vi "Add Compane.vi"(6 "Variant in":variant, 7 "Shift Pressed?":bool, 8 "error in (no error)":errorcluster, 10 "QD Combo Box Ref":refnum<vi>, 11 "QD Launch VI Ref":refnum<vi>) -> (0 "error out":errorcluster, 4 "Variant out":variant)   [LabVIEW 2015]
doc: "Add Control terminal to conpane.\n\nDefault Shortcut - [G]"
uses:
  <vilib>/Utility/config.llb/Read Key (String).vi
  <vilib>/Utility/config.llb/NI_LVConfig.lvlib
panel:
  # "Do not change the connector pane of this VI.\n\nSee the block diagram for directions on how to use this template."
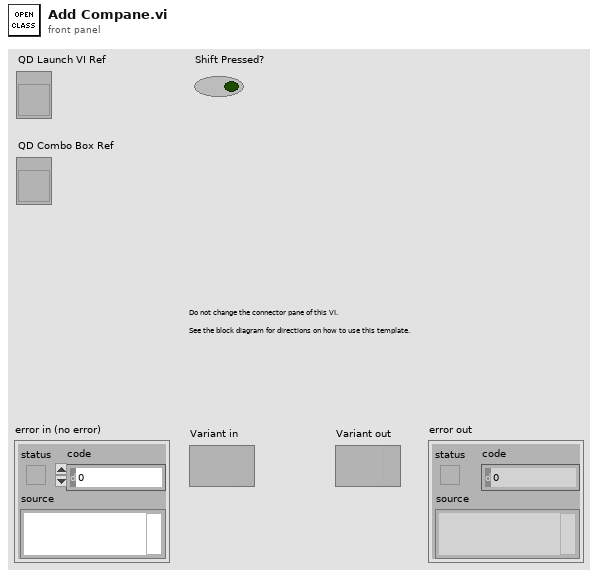
[diagram p1: front panel]
types:
  T1 = typedef "NI_LVConfig.lvlib/Config Data RefNum.ctl" = refnum<k1>
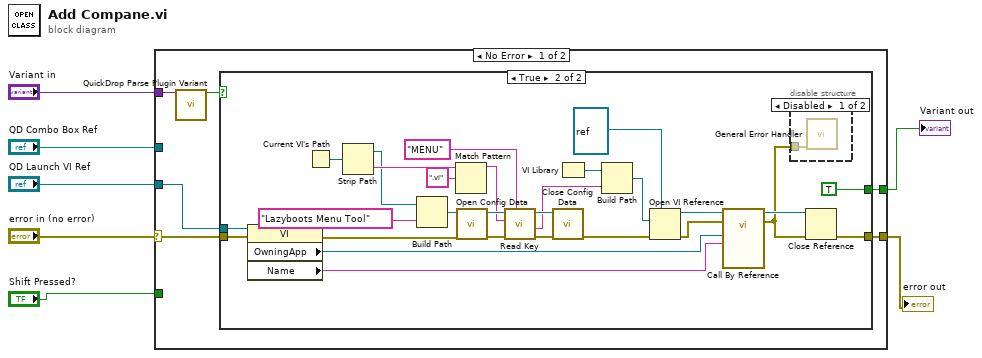
[diagram p0: block diagram]
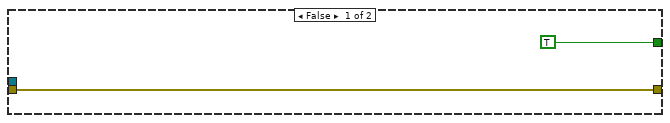
[diagram p2: hidden frame]
diagram:
  n1 = case shown="No Error" "error in (no error)" {
    selector: "error in (no error)" -> [w13 w45]
    tunnel: [w12 w45] -> w2
    tunnel: "QD Launch VI Ref" -> [w11 _]
    tunnel: [w10 _] -> w1
    tunnel: "Variant in" -> [w9 _]
    tunnel: "QD Combo Box Ref" -> [_ _]
    tunnel: "Shift Pressed?" -> [_ _]
    frame No Error {
      n2 = call <vilib>:"QuickDrop Parse Plugin Variant.vi"("QDKS Variant in"=w9) -> ("QD Launch VI Panel?"=w8:bool)  [unwired: 12 in, 2 out]
      n3 = case shown="True" w8 {
        tunnel: w13 -> [w14 w19]
        tunnel: [w14 w43] -> w12
        tunnel: w11 -> [_ w20]
        tunnel: [TRUE TRUE] -> w10
        frame False {
        }
        frame True {
          n4 = property class="VI"(reference=w20, error in=w19) -> (error out=w18:errorcluster, "OwningApp"=w17:refnum<vi>, "Name"=w16:string)  [unwired: 1 out]
          n5 = Current VI's Path() -> (path=w42:path)
          n6 = Strip Path(path=w42) -> (stripped path=w27:path, name=w34:string)
          n7 = Build Path(base path=w27, name or relative path="Lazyboots Menu Tool") -> (appended path=w40:path)
          n8 = Match Pattern(string=w34, regular expression=".vi") -> (before substring=w33:string)  [unwired: 4 out]
          n9 = call <vilib>:"Open Config Data.vi"("error in (no error)"=w18, "configuration file path"=w40) -> ("error out"=w38:errorcluster, "refnum"=w39:T1)  [unwired: 7 in, 1 out]
          n10 = call-poly <vilib>:"Read Key.vi"("section"="MENU", "error in (no error)"=w38, "key"=w33, "refnum"=w39) -> ("error out"=w35:errorcluster, "value"=w30:string, "refnum out"=w36:T1)  [unwired: 2 in, 3 out]
          n11 = call <vilib>:"Close Config Data.vi"("error in (no error)"=w35, "refnum"=w36) -> ("error out"=w28:errorcluster)  [unwired: 1 in, 8 out]
          n12 = VI Library() -> (path=w29:path)
          n13 = Build Path(base path=w29, name or relative path=w30) -> (appended path=w31:path)
          n14 = Open VI Reference(type specifier VI Refnum (for type only)=refnum<vi> refnum, vi path=w31, error in (no error)=w28) -> (vi reference=w24:refnum<vi>, error out=w23:errorcluster)  [unwired: 3 out]
          n15 = call-by-ref "?"(reference=w24, error in=w23, "VI Path"=w16, "Application Reference"=w17) -> (reference out=w22:refnum<vi>, error out=w21:errorcluster)  [unwired: 9 in, 1 out]
          n16 = disable-structure shown="Disabled" {
            disable-tunnel: w21 -> [w44 _]
            frame Disabled {
              n17 = call <vilib>:"General Error Handler.vi"("error in (no error)"=w44) -> ()  [unwired: 10 in, 5 out]
            }
            frame Enabled {
            }
          }
          n18 = Close Reference(reference=w22, error in (no error)=w21) -> (error out=w43:errorcluster)
        }
      }
    }
    frame Error {
    }
  }
  "error out" <- w2
  "Variant out" <- w1
